vi "FPGA main.vi"() -> ()   [LabVIEW 2018]
doc: "This VI shows an example of how to implement a closed loop position move using the NI 9505. The position loop is implemented using PID. The output of the loop is used as the command for the current loop, which then sets the PWM duty cycle for the motor. This example assumes that an encoder is connected for position and velocity feedback. This example does not implement advanced motion features such as trajectory generation and splining."
uses:
  <vilib>/LabVIEW Targets/FPGA/cRIO/cRIO-9505/controls.llb/_nicrio_cRIO-9505_DriveStatus.ctl
  <vilib>/Platform/TimedLoop/XDataNode/timing_clust.ctl
  <vilib>/Platform/TimedLoop/XDataNode/nitl_modes.ctl
  <vilib>/Platform/TimedLoop/XDataNode/wakeup.ctl
  <vilib>/LabVIEW Targets/FPGA/cRIO/cRIO-9505/controls.llb/_nicrio_cRIO-9505_DriveDirection.ctl
  <vilib>/rvi/Emulation/niFpgaGetClockAttributes.vi
  <vilib>/rvi/Emulation/niFpgaSctlEmulationGetInTimedLoop.vi
  <vilib>/rvi/Emulation/niFpgaEmulationReportErrorSimple.vi
  <vilib>/rvi/eio/common/nirviEmuTemplateMethod_errors.vi
  <vilib>/rvi/eio/common/nirviEmuTemplatePropertyGet_noerrors.vi
  <vilib>/rvi/Emulation/niFpgaCriticalErrorInLSC.vi
  <vilib>/rvi/Emulation/niFpgaProcessEmulError.vi
  Instance           4 55Saved   Position Control (closed loop) - NI 9505 (FPGA) .vi
  FGPAGlobals.vi
  Instance           3 55Saved   Position Control (closed loop) - NI 9505 (FPGA) .vi
  <vilib>/eio/EIOMethodNode/EIOMethodNode.xnode
  <vilib>/eio/EIOPropertyNode/EIOPropertyNode.xnode
  <vilib>/Platform/TimedLoop/XDataNode/XDataNode.xnode
  <vilib>/eio/EIONode/EIONode.xnode
  <vilib>/Platform/TimedLoop/XDataNode/XDNodeRunTimeDep.lvlib
  <vilib>/rvi/eio/common/nirviEmuTemplatePropertyGet_errors.vi
  <vilib>/rvi/eio/common/nirviEmuTemplatePropertySet_errors.vi
  <vilib>/rvi/eio/common/nirviEmuTemplatePropertySet_noerrors.vi
panel:
  in  "pwm count 2":i16=2000 caption="PWM rate 2"
  in  "pwm count 1":i16=2000 caption="PWM rate 1"
  in  "manual pwm":bool caption="Manul PWM"
  in  "motor 2":i16 caption="PWM 2"
  in  "motor 1":i16 caption="PWM 1"
  in  "new mode 2":bool caption="Start new\nmode 2"
  in  "new mode":bool caption="Start new\nmode 1"
  in  "Position / Current mode 2":bool=TRUE caption="Position /\nCurrent mode 2"
  in  "Position / Current mode":bool=TRUE caption="Position /\nCurrent mode 1"
  in  "Ipmax":i16=5
  in  "Position Setpoint 2":i32 caption="Encoder 2 setpoint"
  in  "Ki":fxp<+/-,16,10>=0.046875 caption="Ipos"
  in  "Kd":fxp<+/-,16,10>=0.5 caption="Dpos"
  in  "Kp":fxp<+/-,16,10>=0.203125 caption="Ppos"
  in  "Position Loop period (usec)":u16=1000 caption="Loop rate"
  in  "Position Setpoint":i32 caption="Encoder 1 setpoint"
  out "Encoder Position 2":i32 caption="Encoder 2 Position"
  out "Encoder Position":i32 caption="Encoder 1 Position"
  in  "Current Min":i16=11 caption="Min\nCurrent"
  in  "Imax":i16=30000
  in  "Icurrent":fxp<+/-,16,4>=0.050048828125 format="%#_3g"
  in  "Pcurrent":fxp<+/-,16,8>=4.0
  in  "Current Limit":i16=500 caption="Max\nCurrent"
  in  "Current Loop Rate":u32=100 caption="Loop\nRate"
  out "Current Feedback 2":i16 caption="Actual\nCurrent 2"
  out "Current Loop Output 2":i16 caption="PWM\nOutput 2"
  in  "Current Command 2":i16 caption="Desired\nCurrent 2"
  out "Current Feedback":i16 caption="Actual\nCurrent 1"
  out "Current Loop Output":i16 caption="PWM\nOutput 1"
  in  "Current Command":i16 caption="Desired\nCurrent 1"
  out "Solenoid open":bool
  in  "Start reward":bool
  in  "Reward":u32
  out "Licking":bool
  out "Frame counter 2":i16
  out "Frame counter":i16
  out "Drive Status 2":T1=enum."Disabled" caption="Drive 2 Status"
  out "Drive Status":T1=enum."Disabled" caption="Drive 1 Status"
  in  "Enable\nDrives":bool caption="Enable Drives"
  in  "Disable\nDrives":bool caption="Disable Drives"
  # "PWM Generators"
  # "Position Controllers"
  # "Torque Controllers"
  # "Drive Status"
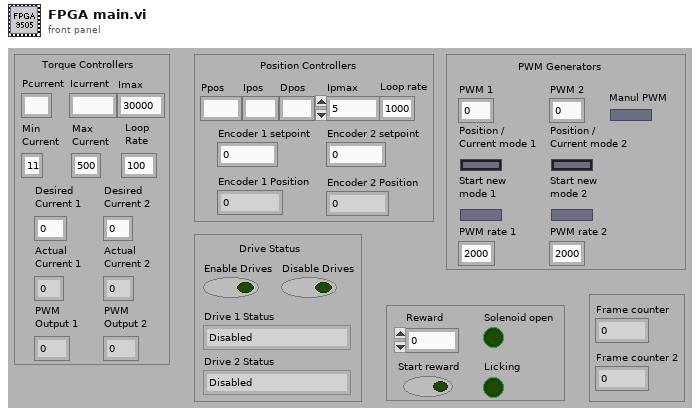
[diagram p1: front panel]
types:
  T1 = typedef "_nicrio_cRIO-9505_DriveStatus.ctl" = enum8{"Enabled", "Disabled", "Disabled by Drive Fault", "Disabled by Temp. Fault", "Disabled by E-Stop", "Unknown"}
  T2 = typedef "XDNodeRunTimeDep.lvlib/timing_clust.ctl" = cluster{"Expected End [f-1]":u64, "Actual End [f-1]":u64, "Finished Late? [f-1]":bool, "Expected End [i-1]":u64, "Actual End [i-1]":u64, "Finished Late? [i-1]":bool, "Expected Start [i]":u64, "Actual Start [i]":u64, "Expected Start [f]":u64, "Actual Start [f]":u64, "Source Name":string, "Structure Name":string, "Period":i64, "Deadline":i64, "Offset":i64, "Start":i64, "Priority":i32, "Timeout":i32, "Mode":T3, "Wakeup Reason":T4, "Error":errorcluster, "Source Type":string, "Secondary Source Type":string, "Global End Time":u64, "Global Start Time":u64, "Frame Duration":u64, "Iteration Duration":u64, "Assigned CPU":i32, "I/O Scan Engine Mode":u32}
  T3 = typedef "XDNodeRunTimeDep.lvlib/nitl_modes.ctl" = enum32{"No Change", "Process missed periods, maintain original phase", "Discard missed periods, maintain original phase", "Process missed periods, ignore original phase", "Discard missed periods, ignore original phase"}
  T4 = typedef "XDNodeRunTimeDep.lvlib/wakeup.ctl" = enum32{"Normal", "Aborted", "Asynchronous wakeup", "Timing source error", "Timed loop error", "Timeout"}
  T5 = typedef "_nicrio_cRIO-9505_DriveDirection.ctl" = enum8{"Clockwise", "Counterclockwise"}
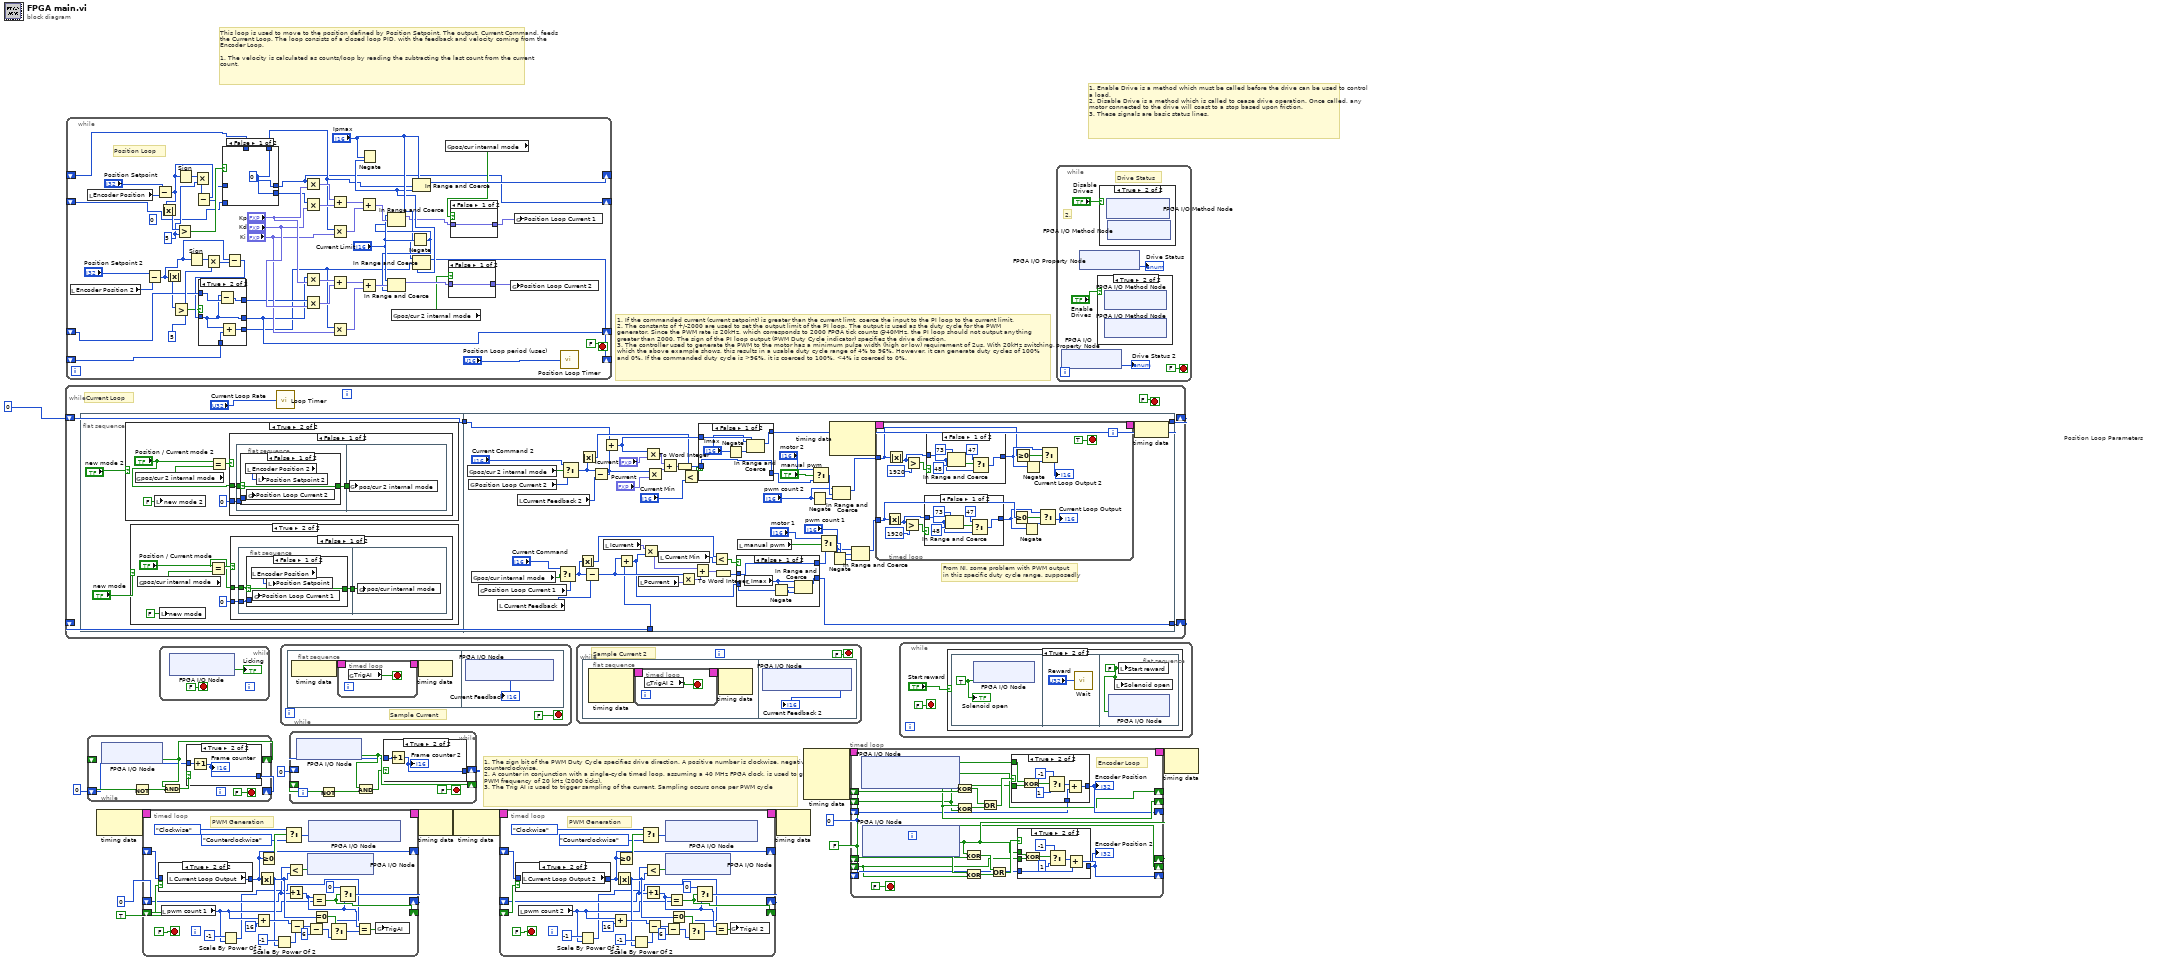
[diagram p0: block diagram]
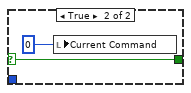
[diagram p10: hidden frame]
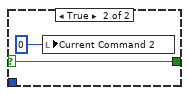
[diagram p13: hidden frame]
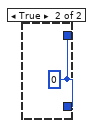
[diagram p15: hidden frame]
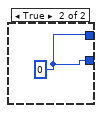
[diagram p16: hidden frame]
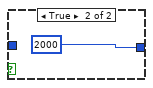
[diagram p17: hidden frame]
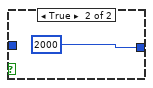
[diagram p18: hidden frame]
diagram:
  w3 = 0 ("Reset Position Value")
  w11 = FALSE ("Encoder Phase A")
  # "Position Loop Parameters"
  # "1. Enable Drive is a method which must be called before the drive can be used to control a load.\n2. Disable Drive is a method which is called to cease drive operation. Once called, any motor connected to the drive will coast to a stop based upon friction.\n3. These signals are basic status lines."
  # "This loop is used to move to the position defined by Position Setpoint. The output, Current Command, feeds the Current Loop. The loop consists of a closed loop PID, with the feedback and velocity coming from the Encoder Loop.\n\n1. The velocity is calculated as counts/loop by reading the subtracting the last count from the current count."
  # "1. The sign bit of the PWM Duty Cycle specifies drive direction. A positive number is clockwise, negative is counterclockwise. \n2. A counter in conjunction with a single-cycle timed loop, assuming a 40 MHz FPGA clock, is used to generate a PWM frequency of 20 kHz (2000 ticks).\n3. The Trig AI is used to trigger sampling of the current. Sampling occurs once per PWM cycle"
  # "1. If the commanded current (current setpoint) is greater than the current limt, coerce the input to the PI loop to the current limit.\n2. The constants of +/-2000 are used to set the output limit of the PI loop. The output is used as the duty cycle for the PWM\ngenerator. Since the PWM rate is 20kHz, which corresponds to 2000 FPGA tick counts @40MHz, the PI loop should not output anything\ngreater than 2000. The sign of the PI loop output (PWM Duty Cycle indicator) specifies the drive direction.\n3. The controller used to generate the PWM to the motor has a minimum pulse width (high or low) requirement of 2us. With 20kHz switching,\nwhich the above example shows, this results in a usable duty cycle range of 4% to 96%. However, it can generate duty cycles of 100%\nand 0%. If the commanded duty cycle is >96%, it is coerced to 100%, <4% is coerced to 0%."
  n1 = while {
    shift-right: [w17] -> _
    shift-left: i16 0 -> [w18]
    shift-right: [w16] -> _
    shift-left: _ -> [w14]
    stop <- FALSE stop-if-true
    # "Current Loop"
    n2 = flat-sequence {
      tunnel: w18 -> [w62]
      tunnel: [w89] -> w17
      tunnel: [w77] -> w16
      tunnel: w14 -> [w63]
      frame #0 {
        n3 = case shown="True" "new mode 2" {
          frame False {
          }
          frame True {
            n4 = global read "FGPAGlobals.vi" "pos/cur 2 internal mode"() -> (w43:bool)
            n5 = local write "new mode 2"(FALSE) -> ()
            n6 = Equal?(x="Position / Current mode 2", y=w43) -> (x = y?=w42:bool)
            n7 = case shown="False" w42 {
              tunnel: "Position / Current mode 2" -> [w46 _]
              tunnel: i16 0 -> [w44 _]
              frame False {
                n8 = flat-sequence {
                  tunnel: w46 -> [w49]
                  tunnel: [w48] -> w45
                  tunnel: w44 -> [w47]
                  tunnel: w45 -> [w55]
                  frame #0 {
                    n9 = case shown="False" w49 {
                      selector: w49 -> [w52 w54]
                      tunnel: [w52 w54] -> w48
                      tunnel: w47 -> [w50 _]
                      frame False {
                        n10 = local read "Encoder Position 2"() -> (w51:i32)
                        n11 = global write "FGPAGlobals.vi" "Position Loop Current 2"(w50) -> ()
                        n12 = local write "Position Setpoint 2"(w51) -> ()
                      }
                      frame True {
                        n13 = local write "Current Command 2"(i16 0) -> ()
                      }
                    }
                  }
                  frame #1 {
                    n14 = global write "FGPAGlobals.vi" "pos/cur 2 internal mode"(w55) -> ()
                  }
                }
              }
              frame True {
              }
            }
          }
        }
        n15 = case shown="True" "new mode" {
          frame False {
          }
          frame True {
            n16 = global read "FGPAGlobals.vi" "pos/cur internal mode"() -> (w25:bool)
            n17 = local write "new mode"(FALSE) -> ()
            n18 = Equal?(x="Position / Current mode", y=w25) -> (x = y?=w24:bool)
            n19 = case shown="False" w24 {
              tunnel: "Position / Current mode" -> [w29 _]
              tunnel: i16 0 -> [w27 _]
              frame False {
                n20 = flat-sequence {
                  tunnel: w29 -> [w32]
                  tunnel: [w31] -> w28
                  tunnel: w27 -> [w30]
                  tunnel: w28 -> [w38]
                  frame #0 {
                    n21 = case shown="False" w32 {
                      selector: w32 -> [w35 w37]
                      tunnel: [w35 w37] -> w31
                      tunnel: w30 -> [w33 _]
                      frame False {
                        n22 = local read "Encoder Position"() -> (w34:i32)
                        n23 = global write "FGPAGlobals.vi" "Position Loop Current 1"(w33) -> ()
                        n24 = local write "Position Setpoint"(w34) -> ()
                      }
                      frame True {
                        n25 = local write "Current Command"(i16 0) -> ()
                      }
                    }
                  }
                  frame #1 {
                    n26 = global write "FGPAGlobals.vi" "pos/cur internal mode"(w38) -> ()
                  }
                }
              }
              frame True {
              }
            }
          }
        }
      }
      frame #1 {
        # "From NI, some problem with PWM output\nin this specific duty cycle range, supposedly"
        n27 = global read "FGPAGlobals.vi" "pos/cur 2 internal mode"() -> (w75:bool)
        n28 = global read "FGPAGlobals.vi" "Position Loop Current 2"() -> (w76:i16)
        n29 = global read "FGPAGlobals.vi" "pos/cur internal mode"() -> (w74:bool)
        n30 = global read "FGPAGlobals.vi" "Position Loop Current 1"() -> (w105:i16)
        n31 = local read "Current Feedback"() -> (w97:i16)
        n32 = local read "Current Feedback 2"() -> (w102:i16)
        n33 = Select(t="Current Command", s=w74, f=w105) -> (s? t:f=w64:i16)
        n34 = Select(t="Current Command 2", s=w75, f=w76) -> (s? t:f=w69:i16)
        n35 = Absolute Value(x=w64) -> (abs(x)=w79:i16)
        n36 = Absolute Value(x=w69) -> (abs(x)=w82:i16)
        n37 = Subtract(x=w64, y=w97) -> (x-y=w96:i16)
        n38 = Subtract(x=w69, y=w102) -> (x-y=w101:i16)
        n39 = Add(x=w62, y=w101) -> (x+y=w90:i16)
        n40 = local read "Icurrent"() -> (w67:fxp<+/-,16,4>)
        n41 = Add(x=w96, y=w63) -> (x+y=w88:i16)
        n42 = local read "Pcurrent"() -> (w68:fxp<+/-,16,8>)
        n43 = Multiply(x=w67, y=w88) -> (x*y=w93:fxp<+/-,32,20>)
        n44 = Multiply(x=w90, y="Icurrent") -> (x*y=w100:fxp<+/-,32,20>)
        n45 = Multiply(x=w101, y="Pcurrent") -> (x*y=w99:fxp<+/-,32,24>)
        n46 = local read "Current Min"() -> (w66:i16)
        n47 = Add(x=w100, y=w99) -> (x+y=w81:fxp<+/-,36,24>)
        n48 = To Word Integer(number=w81) -> (16bit integer=w58:i16)
        n49 = Multiply(x=w96, y=w68) -> (x*y=w94:fxp<+/-,32,24>)
        n50 = Less?(x=w82, y="Current Min") -> (x < y?=w59:bool)
        n51 = Add(x=w93, y=w94) -> (x+y=w80:fxp<+/-,36,24>)
        n52 = case shown="False" w59 {
          tunnel: w90 -> [w112 _]
          tunnel: [w111 w113] -> w89
          tunnel: w58 -> [w108 _]
          tunnel: [w108 w113] -> w57
          frame False {
            n53 = Negate(x="Imax") -> (-x=w109:i16)
            n54 = In Range and Coerce(upper limit="Imax", x=w112, lower limit=w109) -> (coerced(x)=w111:i16)  [unwired: 1 out]
          }
          frame True {
            w113 = i16 0 ("lower limit")
          }
        }
        n55 = Less?(x=w79, y=w66) -> (x < y?=w61:bool)
        n56 = To Word Integer(number=w80) -> (16bit integer=w60:i16)
        n57 = case shown="False" w61 {
          tunnel: w88 -> [w118 _]
          tunnel: [w117 w119] -> w77
          tunnel: [w114 w119] -> w56
          tunnel: w60 -> [w114 _]
          frame False {
            n58 = local read "Imax"() -> (w116:i16)
            n59 = Negate(x=w116) -> (-x=w115:i16)
            n60 = In Range and Coerce(upper limit=w116, x=w118, lower limit=w115) -> (coerced(x)=w117:i16)  [unwired: 1 out]
          }
          frame True {
            w119 = i16 0
          }
        }
        n61 = local read "manual pwm"() -> (w65:bool)
        n62 = Negate(x="pwm count 2") -> (-x=w71:i16)
        n63 = Select(t="motor 2", s="manual pwm", f=w57) -> (s? t:f=w84:i16)
        n64 = Select(t="motor 1", s=w65, f=w56) -> (s? t:f=w85:i16)
        n65 = node-c288() -> (w107:T2)  [unwired: 2 out]
        n66 = Negate(x="pwm count 1") -> (-x=w70:i16)
        n67 = In Range and Coerce(upper limit="pwm count 2", x=w84, lower limit=w71) -> (coerced(x)=w98:i16)  [unwired: 1 out]
        n68 = In Range and Coerce(upper limit="pwm count 1", x=w85, lower limit=w70) -> (coerced(x)=w91:i16)  [unwired: 1 out]
        n69 = timed-loop {
          timing: w107 -> [_]
          timing-out: [_] -> w106
          tunnel: w98 -> [w121]
          tunnel: w91 -> [w129]
          stop <- TRUE stop-if-true
          n70 = Absolute Value(x=w129) -> (abs(x)=w130:i16)
          n71 = Absolute Value(x=w121) -> (abs(x)=w126:i16)
          n72 = Greater?(x=w130, y=i16 1920 ("upper limit")) -> (0:w131:bool)
          n73 = Greater?(x=w126, y=i16 1920 ("upper limit")) -> (0:w125:bool)
          n74 = case shown="False" w131 {
            tunnel: w130 -> [w145 _]
            tunnel: [w144 i16 2000 ("upper limit")] -> w128
            frame False {
              n75 = In Range and Coerce(upper limit=i16 73 ("lower limit"), x=w145, lower limit=i16 48) -> (In Range?=w147:bool)  [unwired: 1 out]
              n76 = Select(t=i16 47 ("lower limit"), s=w147, f=w145) -> (s? t:f=w144:i16)
            }
            frame True {
            }
          }
          n77 = case shown="False" w125 {
            tunnel: w126 -> [w138 _]
            tunnel: [w137 i16 2000 ("upper limit")] -> w127
            frame False {
              n78 = In Range and Coerce(upper limit=i16 73 ("lower limit"), x=w138, lower limit=i16 48) -> (In Range?=w140:bool)  [unwired: 1 out]
              n79 = Select(t=i16 47 ("lower limit"), s=w140, f=w138) -> (s? t:f=w137:i16)
            }
            frame True {
            }
          }
          n80 = Greater Or Equal To 0?(x=w129) -> (x >= 0?=w136:bool)
          n81 = Greater Or Equal To 0?(x=w121) -> (x >= 0?=w122:bool)
          n82 = Negate(x=w128) -> (-x=w135:i16)
          n83 = Negate(x=w127) -> (-x=w123:i16)
          n84 = Select(t=w128, s=w136, f=w135) -> (s? t:f=→"Current Loop Output":i16)
          n85 = Select(t=w127, s=w122, f=w123) -> (s? t:f=→"Current Loop Output 2":i16)
        }
        n86 = node-c288(w106) -> ()
      }
    }
    n87 = call "Loop Timer"("Count(uSec)"="Current Loop Rate") -> ()  [unwired: 1 out]
  }
  n88 = while "Position Control Loop" {
    shift-right: [w164] -> _
    shift-left: _ -> [w165]
    shift-right: [w160] -> _
    shift-left: _ -> [w163]
    shift-right: [w185] -> _
    shift-left: _ -> [w158]
    shift-right: [w188] -> _
    shift-left: _ -> [w167]
    stop <- FALSE stop-if-true
    w176 = 5
    w174 = 5
    (unwired) 0
    # "Position Loop"
    n89 = local read "Encoder Position 2"() -> (w191:i32)
    n90 = local read "Encoder Position"() -> (w206:i32)
    n91 = Subtract(x="Position Setpoint 2", y=w191) -> (x-y=w157:i32)
    n92 = Subtract(x="Position Setpoint", y=w206) -> (x-y=w171:i32)
    n93 = Absolute Value(x=w171) -> (abs(x)=w178:i32)
    n94 = Absolute Value(x=w157) -> (abs(x)=w162:i32)
    n95 = Greater?(x=w162, y=w176) -> (0:w155:bool)
    n96 = Greater?(x=w178, y=w174) -> (0:w170:bool)
    n97 = Sign(1:w171) -> (0:w173:i32)
    n98 = Sign(1:w157) -> (0:w177:i32)
    n99 = Multiply(x=w173, y=w174) -> (x*y=w172:i32)
    n100 = Subtract(x=w171, y=w172) -> (x-y=w169:i32)
    n101 = Multiply(x=w177, y=w176) -> (x*y=w175:i32)
    n102 = case shown="False" w170 {
      tunnel: w169 -> [_ w219]
      tunnel: [w216 w219] -> w164
      tunnel: [w216 w221] -> w168
      tunnel: w167 -> [_ w220]
      tunnel: [w216 w218] -> w166
      tunnel: w165 -> [_ w217]
      frame False {
        w216 = 0
      }
      frame True {
        n103 = Subtract(x=w219, y=w217) -> (x-y=w221:i32)
        n104 = Add(x=w220, y=w219) -> (x+y=w218:i32)
      }
    }
    n105 = Subtract(x=w157, y=w175) -> (x-y=w156:i32)
    n106 = case shown="True" w155 {
      tunnel: w163 -> [_ w215]
      tunnel: [w210 w214] -> w161
      tunnel: [w210 w211] -> w160
      tunnel: [w210 w213] -> w159
      tunnel: w158 -> [_ w212]
      tunnel: w156 -> [_ w211]
      frame False {
        w210 = 0
      }
      frame True {
        n107 = Subtract(x=w211, y=w215) -> (x-y=w214:i32)
        n108 = Add(x=w211, y=w212) -> (x+y=w213:i32)
      }
    }
    n109 = Multiply(x=w164, y="Kp") -> (x*y=w205:fxp<+/-,48,42>)
    n110 = Multiply(x=w168, y="Kd") -> (x*y=w204:fxp<+/-,48,42>)
    n111 = Multiply(x=w160, y="Kp") -> (x*y=w200:fxp<+/-,48,42>)
    n112 = Multiply(x=w161, y="Kd") -> (x*y=w199:fxp<+/-,48,42>)
    n113 = Add(x=w205, y=w204) -> (x+y=w203:fxp<+/-,49,43>)
    n114 = Multiply(x=w166, y="Ki") -> (x*y=w202:fxp<+/-,48,42>)
    n115 = Add(x=w200, y=w199) -> (x+y=w198:fxp<+/-,49,43>)
    n116 = Multiply(x=w159, y="Ki") -> (x*y=w197:fxp<+/-,48,42>)
    n117 = Add(x=w203, y=w202) -> (x+y=w201:fxp<+/-,49,43>)
    n118 = Add(x=w198, y=w197) -> (x+y=w196:fxp<+/-,49,43>)
    n119 = Negate(x="Ipmax") -> (-x=w186:i16)
    n120 = global read "FGPAGlobals.vi" "pos/cur 2 internal mode"() -> (w180:bool)
    n121 = Negate(x="Current Limit") -> (-x=w189:i16)
    n122 = In Range and Coerce(upper limit="Current Limit", x=w201, lower limit=w189) -> (coerced(x)=w184:fxp<+/-,49,43>)  [unwired: 1 out]
    n123 = In Range and Coerce(upper limit="Current Limit", x=w196, lower limit=w189) -> (coerced(x)=w182:fxp<+/-,49,43>)  [unwired: 1 out]
    n124 = In Range and Coerce(upper limit="Ipmax", x=w159, lower limit=w186) -> (coerced(x)=w185:i32)  [unwired: 1 out]
    n125 = In Range and Coerce(upper limit="Ipmax", x=w166, lower limit=w186) -> (coerced(x)=w188:i32)  [unwired: 1 out]
    n126 = global read "FGPAGlobals.vi" "pos/cur internal mode"() -> (w179:bool)
    n127 = case shown="False" w180 {
      tunnel: w182 -> [w222 _]
      tunnel: [w222 fxp<+/-,49,43> 0.0] -> w181
      frame False {
      }
      frame True {
      }
    }
    n128 = case shown="False" w179 {
      tunnel: w184 -> [w224 _]
      tunnel: [w224 fxp<+/-,49,43> 0.0] -> w183
      frame False {
      }
      frame True {
      }
    }
    n129 = global write "FGPAGlobals.vi" "Position Loop Current 2"(w181) -> ()
    n130 = global write "FGPAGlobals.vi" "Position Loop Current 1"(w183) -> ()
    n131 = call "Position Loop Timer"("Count(uSec)"="Position Loop period (usec)") -> ()  [unwired: 1 out]
  }
  n132 = while {
    shift-right: [w231] -> _
    shift-left: _ -> [w230]
    shift-right: [w228] -> _
    shift-left: i16 0 -> [w227]
    stop <- FALSE stop-if-true
    n133 = xnode "FPGA I/O Node"() -> ("Mod4/DIO9"=w231:bool)  [unwired: 1 in, 1 out]
    n134 = Not(x=w230) -> (.not. x?=w229:bool)
    n135 = And(x=w231, y=w229) -> (x .and. y?=w226:bool)
    n136 = case shown="True" w226 {
      tunnel: [w233 w234] -> w228
      tunnel: w227 -> [w233 w235]
      frame False {
      }
      frame True {
        n137 = Increment(x=w235) -> (x+1=w234:i16)
        "Frame counter" <- w234
      }
    }
  }
  n138 = node-c288() -> (w10:T2)  [unwired: 1 out]
  n139 = timed-loop {
    timing: w10 -> [_]
    timing-out: [_] -> w9
    shift-right: [w262] -> _
    shift-left: i16 0 -> [w239]
    shift-right: [w261] -> _
    shift-left: TRUE -> [w251]
    shift-right: [w253] -> _
    shift-left: _ -> [w260]
    stop <- FALSE stop-if-true
    # "PWM Generation"
    n140 = case shown="True" w251 {
      tunnel: [w264 w265] -> w253
      tunnel: w260 -> [w264 _]
      frame False {
      }
      frame True {
        n141 = local read "Current Loop Output"() -> (w265:i16)
      }
    }
    n142 = local read "pwm count 1"() -> (w237:i16)
    n143 = Scale By Power Of 2(n=i16 -1, x=w237) -> (x*2^n=w236:i16)
    n144 = Add(x=w237, y=i16 16) -> (x+y=w247:i16)
    n145 = Absolute Value(x=w253) -> (abs(x)=w240:i16)
    n146 = Greater Or Equal To 0?(x=w253) -> (x >= 0?=w259:bool)
    n147 = Scale By Power Of 2(n=i16 -1, x=w240) -> (x*2^n=w248:i16)
    n148 = Select(t=_nicrio_cRIO-9505_DriveDirection."Clockwise" ("Drive Direction"), s=w259, f=_nicrio_cRIO-9505_DriveDirection."Counterclockwise" ("Drive Direction")) -> (s? t:f=w255:T5)
    n149 = Less?(x=w239, y=w240) -> (x < y?=w256:bool)
    n150 = Increment(x=w239) -> (x+1=w243:i16)
    n151 = Subtract(x=w247, y=w248) -> (x-y=w246:i16)
    n152 = Subtract(x=w246, y=i16 6) -> (x-y=w244:i16)
    n153 = xnode "FPGA I/O Node"("Mod1/Motor"=w256) -> ()  [unwired: 1 in, 1 out]
    n154 = xnode "FPGA I/O Node"("Mod1/Drive Direction"=w255) -> ()  [unwired: 1 in, 1 out]
    n155 = Equal?(x=w243, y=w237) -> (x = y?=w261:bool)
    n156 = Equal To 0?(x=w240) -> (x = 0?=w250:bool)
    n157 = Select(t=w236, s=w250, f=w244) -> (s? t:f=w242:i16)
    n158 = Select(t=i16 0, s=w261, f=w243) -> (s? t:f=w262:i16)
    n159 = Equal?(x=w243, y=w242) -> (x = y?=w241:bool)
    n160 = global write "FGPAGlobals.vi" "TrigAI"(w241) -> ()
  }
  n161 = while {
    stop <- FALSE stop-if-true
    n162 = xnode "FPGA I/O Node"() -> ("Mod4/DIO12"=→"Licking":bool)  [unwired: 1 in, 1 out]
  }
  n163 = while {
    stop <- FALSE stop-if-true
    # "Sample Current"
    n164 = flat-sequence {
      frame #0 {
        n165 = node-c288() -> (w272:T2)
        n166 = timed-loop {
          timing: w272 -> [_]
          timing-out: [_] -> w271
          stop <- w273 stop-if-true
          n167 = global read "FGPAGlobals.vi" "TrigAI"() -> (w273:bool)
        }
        n168 = node-c288(w271) -> ()
      }
      frame #1 {
        n169 = xnode "FPGA I/O Node"() -> ("Mod1/Current Sense"=→"Current Feedback":i16)  [unwired: 1 in, 1 out]
      }
    }
  }
  n170 = while {
    shift-right: [w284] -> _
    shift-left: _ -> [w283]
    shift-right: [w281] -> _
    shift-left: i16 0 -> [w280]
    stop <- FALSE stop-if-true
    n171 = xnode "FPGA I/O Node"() -> ("Mod4/DIO10"=w284:bool)  [unwired: 1 in, 1 out]
    n172 = Not(x=w283) -> (.not. x?=w282:bool)
    n173 = And(x=w284, y=w282) -> (x .and. y?=w279:bool)
    n174 = case shown="True" w279 {
      tunnel: [w286 w287] -> w281
      tunnel: w280 -> [w286 w288]
      frame False {
      }
      frame True {
        n175 = Increment(x=w288) -> (x+1=w287:i16)
        "Frame counter 2" <- w287
      }
    }
  }
  n176 = node-c288(w9) -> ()  [unwired: 1 out]
  n177 = node-c288() -> (w2:T2)  [unwired: 1 out]
  n178 = timed-loop {
    timing: w2 -> [_]
    timing-out: [_] -> w1
    shift-right: [w315] -> _
    shift-left: _ -> [w292]
    shift-right: [w314] -> _
    shift-left: _ -> [w304]
    shift-right: [w306] -> _
    shift-left: _ -> [w313]
    stop <- FALSE stop-if-true
    # "PWM Generation"
    n179 = case shown="True" w304 {
      tunnel: [w317 w318] -> w306
      tunnel: w313 -> [w317 _]
      frame False {
      }
      frame True {
        n180 = local read "Current Loop Output 2"() -> (w318:i16)
      }
    }
    n181 = local read "pwm count 2"() -> (w290:i16)
    n182 = Scale By Power Of 2(n=i16 -1, x=w290) -> (x*2^n=w289:i16)
    n183 = Add(x=w290, y=i16 16) -> (x+y=w300:i16)
    n184 = Absolute Value(x=w306) -> (abs(x)=w293:i16)
    n185 = Greater Or Equal To 0?(x=w306) -> (x >= 0?=w312:bool)
    n186 = Scale By Power Of 2(n=i16 -1, x=w293) -> (x*2^n=w301:i16)
    n187 = Select(t=_nicrio_cRIO-9505_DriveDirection."Clockwise" ("Drive Direction"), s=w312, f=_nicrio_cRIO-9505_DriveDirection."Counterclockwise" ("Drive Direction")) -> (s? t:f=w308:T5)
    n188 = Less?(x=w292, y=w293) -> (x < y?=w309:bool)
    n189 = Increment(x=w292) -> (x+1=w296:i16)
    n190 = Subtract(x=w300, y=w301) -> (x-y=w299:i16)
    n191 = Subtract(x=w299, y=i16 6) -> (x-y=w297:i16)
    n192 = xnode "FPGA I/O Node"("Mod2/Motor"=w309) -> ()  [unwired: 1 in, 1 out]
    n193 = xnode "FPGA I/O Node"("Mod2/Drive Direction"=w308) -> ()  [unwired: 1 in, 1 out]
    n194 = Equal?(x=w296, y=w290) -> (x = y?=w314:bool)
    n195 = Equal To 0?(x=w293) -> (x = 0?=w303:bool)
    n196 = Select(t=w289, s=w303, f=w297) -> (s? t:f=w295:i16)
    n197 = Select(t=i16 0, s=w314, f=w296) -> (s? t:f=w315:i16)
    n198 = Equal?(x=w296, y=w295) -> (x = y?=w294:bool)
    n199 = global write "FGPAGlobals.vi" "TrigAI 2"(w294) -> ()
  }
  n200 = while {
    stop <- FALSE stop-if-true
    # "Sample Current 2"
    n201 = flat-sequence {
      frame #0 {
        n202 = node-c288() -> (w323:T2)  [unwired: 1 in, 1 out]
        n203 = timed-loop {
          timing: w323 -> [_]
          timing-out: [_] -> w322
          stop <- w324 stop-if-true
          n204 = global read "FGPAGlobals.vi" "TrigAI 2"() -> (w324:bool)
        }
        n205 = node-c288(w322) -> ()  [unwired: 1 out]
      }
      frame #1 {
        n206 = xnode "FPGA I/O Node"() -> ("Mod2/Current Sense"=→"Current Feedback 2":i16)  [unwired: 1 in, 1 out]
      }
    }
  }
  n207 = node-c288(w1) -> ()  [unwired: 1 out]
  n208 = node-c288() -> (w13:T2)  [unwired: 4 out]
  n209 = timed-loop {
    shift-right: [w341] -> _
    shift-left: w11 -> [w348]
    shift-right: [w343] -> _
    shift-left: w11 -> [w340]
    shift-right: [w342] -> _
    shift-left: w3 -> [w339]
    timing: w13 -> [_]
    timing-out: [_] -> w12
    shift-right: [w335] -> _
    shift-left: w11 -> [w330]
    shift-right: [w334] -> _
    shift-left: w11 -> [w331]
    shift-right: [w333] -> _
    shift-left: w3 -> [w332]
    stop <- FALSE stop-if-true
    # "Encoder Loop"
    n210 = xnode "FPGA I/O Node"() -> ("Mod1/Encoder Phase A"=w341:bool, "Mod1/Encoder Phase B"=w343:bool)  [unwired: 2 in, 2 out]
    n211 = xnode "FPGA I/O Node"() -> ("Mod2/Encoder Phase A"=w335:bool, "Mod2/Encoder Phase B"=w334:bool)  [unwired: 2 in, 2 out]
    n212 = Exclusive Or(1:w348, 2:w341) -> (0:w347:bool)
    n213 = Exclusive Or(1:w340, 2:w343) -> (0:w346:bool)
    n214 = Exclusive Or(1:w330, 2:w335) -> (0:w338:bool)
    n215 = Exclusive Or(1:w331, 2:w334) -> (0:w337:bool)
    n216 = Or(x=w347, y=w346) -> (x .or. y?=w345:bool)
    n217 = Or(x=w338, y=w337) -> (x .or. y?=w336:bool)
    n218 = case shown="True" w345 {
      tunnel: [w358 w364] -> w342
      tunnel: w341 -> [_ w366]
      tunnel: w340 -> [_ w365]
      tunnel: w339 -> [w358 w363]
      frame False {
      }
      frame True {
        n219 = Exclusive Or(1:w365, 2:w366) -> (0:w359:bool)
        n220 = Select(t=-1, s=w359, f=1) -> (s? t:f=w360:i32)
        n221 = Add(x=w360, y=w363) -> (x+y=w364:i32)
      }
    }
    "Encoder Position" <- w342
    n222 = case shown="True" w336 {
      tunnel: w335 -> [_ w357]
      tunnel: w331 -> [_ w356]
      tunnel: w332 -> [w349 w354]
      tunnel: [w349 w355] -> w333
      frame False {
      }
      frame True {
        n223 = Exclusive Or(1:w356, 2:w357) -> (0:w352:bool)
        n224 = Select(t=-1, s=w352, f=1) -> (s? t:f=w351:i32)
        n225 = Add(x=w351, y=w354) -> (x+y=w355:i32)
      }
    }
    "Encoder Position 2" <- w333
  }
  n226 = while {
    stop <- FALSE stop-if-true
    n227 = case shown="True" "Start reward" {
      frame False {
      }
      frame True {
        n228 = flat-sequence {
          frame #0 {
            w371 = TRUE
            n229 = xnode "FPGA I/O Node"("Mod4/DIO6"=w371) -> ()  [unwired: 1 in, 1 out]
            "Solenoid open" <- w371
          }
          frame #1 {
            n230 = call "Wait"("Count(mSec)"="Reward") -> ()  [unwired: 1 out]
          }
          frame #2 {
            w373 = FALSE
            n231 = xnode "FPGA I/O Node"("Mod4/DIO6"=w373) -> ()  [unwired: 1 in, 1 out]
            n232 = local write "Solenoid open"(w373) -> ()
            n233 = local write "Start reward"(w373) -> ()
          }
        }
      }
    }
  }
  n234 = while {
    stop <- FALSE stop-if-true
    # "Drive Status"
    # "2."
    n235 = xnode "FPGA I/O Property Node"() -> ("Drive Status"=→"Drive Status 2":T1)  [unwired: 1 in, 1 out]
    n236 = xnode "FPGA I/O Property Node"() -> ("Drive Status"=→"Drive Status":T1)  [unwired: 1 in, 1 out]
    n237 = case shown="True" "Enable\nDrives" {
      frame False {
      }
      frame True {
        n238 = xnode "FPGA I/O Method Node"() -> ()  [unwired: 1 in, 1 out]
        n239 = xnode "FPGA I/O Method Node"() -> ()  [unwired: 1 in, 1 out]
      }
    }
    n240 = case shown="True" "Disable\nDrives" {
      frame False {
      }
      frame True {
        n241 = xnode "FPGA I/O Method Node"() -> ()  [unwired: 1 in, 1 out]
        n242 = xnode "FPGA I/O Method Node"() -> ()  [unwired: 1 in, 1 out]
      }
    }
  }
  n243 = node-c288(w12) -> ()  [unwired: 1 out]
